vi "R1KSignalProcess.vi"(9 "error":errorcluster, 11 "LabVIEW Web Service":refnum<class "Web Service.lvclass">) -> (1 "error out":errorcluster)   [LabVIEW 2016]
uses:
  <vilib>/wsapi/Web Service.lvclass
  Controls/ISE.ctl
  Controls/Tri State Control.ctl
  Controls/ISE_CF.ctl
panel:
  out "R1Na":T1 {"Steady State?" items=["False", "True", "NaN", ""]}
  out "Carousel Array":dbl[][](array[numeric])
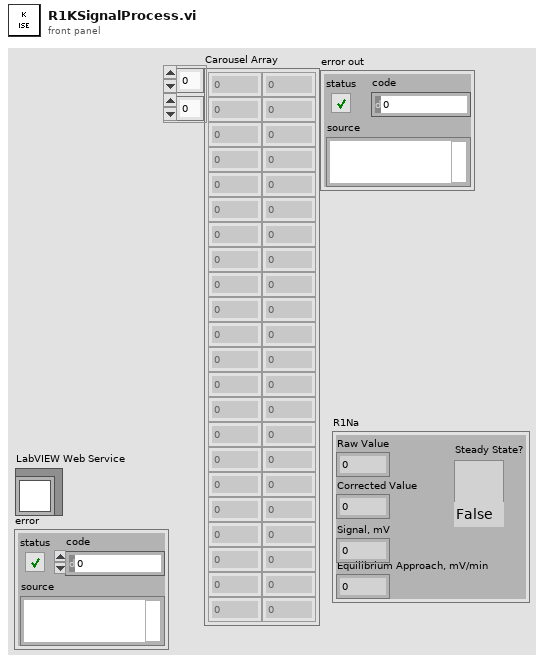
[diagram p1: front panel]
types:
  T1 = typedef "ISE.ctl" = cluster{"Raw Value":dbl, "Corrected Value":dbl, "Signal, mV":dbl, "Equilibrium Approach, mV/min":dbl, "Steady State?":T2}
  T2 = typedef "Tri State Control.ctl" = u16
  T3 = typedef "ISE_CF.ctl" = cluster{"Correction Factor":dbl, "Ion":string, "Correct For Ion?":bool}
  T4 = cluster{"Equil Approach Set point, mV/min":dbl, "Equil Approach dt, s":dbl, "Interference Correction Factors":T3[], "Detect Equilibrium?":bool, "Probe Intercept":dbl, "Probe Slope":dbl, "Baseline":dbl, "Detection Limit, M":dbl}
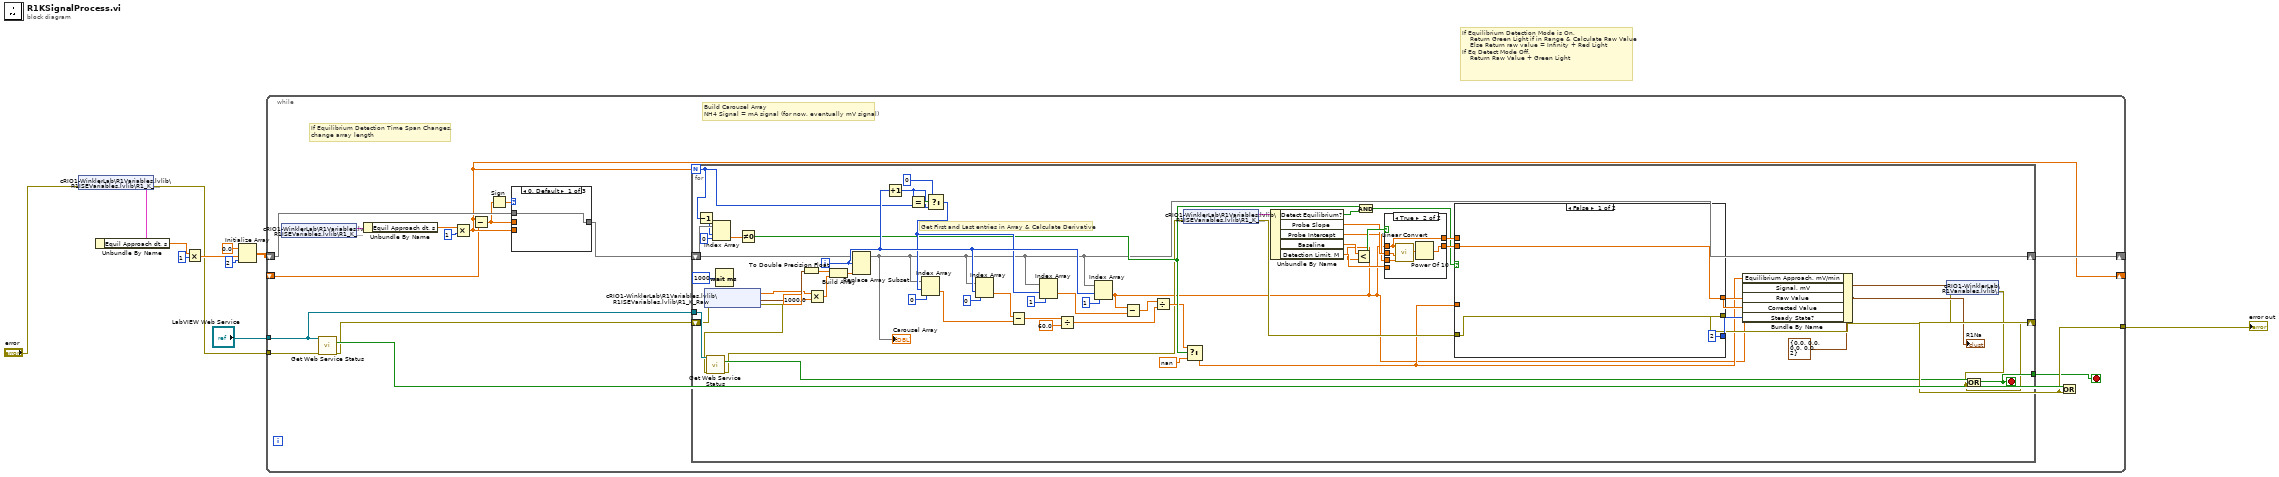
[diagram p0: block diagram]
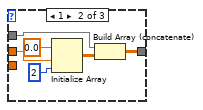
[diagram p2: hidden frame]
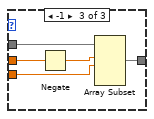
[diagram p3: hidden frame]
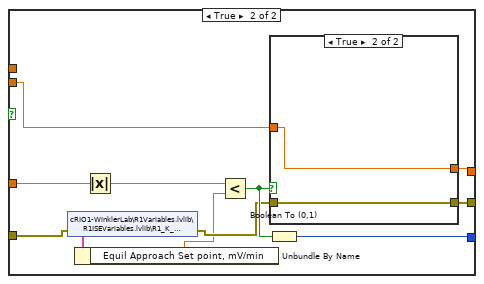
[diagram p5: hidden frame]
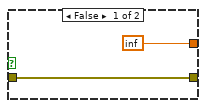
[diagram p6: hidden frame]
diagram:
  # "If Equilibrium Detection Mode is On, \n    Return Green Light if in Range & Calculate Raw Value\n    Else Return raw value = Infinity + Red Light\nIf Eq Detect Mode Off,\n    Return Raw Value + Green Light"
  n1 = shared-variable "cRIO1-WinklerLab\\R1Variables.lvlib\\R1ISEVariables.lvlib\\R1_K_SetParams"(error in="error") -> (w5:T4, error out=w1:errorcluster)
  n2 = Unbundle By Name(w5) -> ("Equil Approach dt, s"=w4:dbl)
  n3 = Multiply(x=w4, y=1) -> (x*y=w3:dbl)
  n4 = Initialize Array(0.0 ("element"), w3, 2 ("dimension size")) -> (w7:dbl[][])
  n5 = while {
    tunnel: "LabVIEW Web Service" -> [w27]
    tunnel: w1 -> [w17]
    shift-right: [w21] -> _
    shift-left: w7 -> [w24]
    shift-right: [w20] -> _
    shift-left: _ -> [w19]
    tunnel: [w16] -> w6
    stop <- w15 stop-if-true
    # "Build Carousel Array\nNH4 Signal = mA signal (for now, eventually mV signal)"
    # "If Equilibrium Detection Time Span Changes, \nchange array length"
    n6 = shared-variable "cRIO1-WinklerLab\\R1Variables.lvlib\\R1ISEVariables.lvlib\\R1_K_SetParams"() -> (w13:T4)  [unwired: 1 in, 1 out]
    n7 = call <vilib>:"Get Web Service Status.vi"("LabVIEW Web Service"=w27, "error in (no error)"=w17) -> ("service stopping?"=w18:bool, "error out"=w14:errorcluster)  [unwired: 11 in, 1 out]
    n8 = Unbundle By Name(w13) -> ("Equil Approach dt, s"=w12:dbl)
    n9 = Multiply(x=w12, y=1) -> (x*y=w20:dbl)
    n10 = Subtract(x=w20, y=w19) -> (x-y=w23:dbl)
    n11 = Sign(1:w23) -> (0:w25:dbl)
    n12 = case shown="0, Default" w25 {
      tunnel: w24 -> [w28 w32 w35]
      tunnel: w23 -> [_ w29 w37]
      tunnel: [w28 w30 w39] -> w22
      tunnel: w20 -> [_ _ w38]
      frame 0, Default {
      }
      frame 1 {
        n13 = Initialize Array(0.0 ("element"), w29, 2 ("dimension size")) -> (w31:dbl[][])
        n14 = Build Array (concatenate)(w32, w31) -> (w30:dbl[][])
      }
      frame -1 {
        n15 = Negate(x=w37) -> (-x=w36:dbl)
        n16 = Array Subset(array=w35, index (row)=w36, length (row)=w38) -> (w39:dbl[][])  [unwired: 2 in]
      }
    }
    n17 = for {
      N: w20 -> [w74]
      tunnel: w27 -> [w96]
      shift-right: [w68] -> w21
      shift-left: w22 -> [w80]
      shift-right: [w57] -> w16
      shift-left: w14 -> [w61]
      tunnel: [w60] -> w15
      i -> [w85]
      stop <- w60 stop-if-true
      # "Get First and Last entries in Array & Calculate Derivative"
      n18 = Decrement(x=w74) -> (x-1=w75:i32)
      n19 = shared-variable "cRIO1-WinklerLab\\R1Variables.lvlib\\R1ISEVariables.lvlib\\R1_K_Raw"(error in=w61) -> (w51:dbl, error out=w71:errorcluster, w72:timestamp)
      n20 = call <vilib>:"Get Web Service Status.vi"("LabVIEW Web Service"=w96, "error in (no error)"=w71) -> ("service stopping?"=w73:bool, "error out"=w56:errorcluster)  [unwired: 11 in, 1 out]
      n21 = Index Array(array=w80, index (row)=w75, index (col)=0 ("disabled index (col)")) -> (element=w78:dbl)
      n22 = Wait (ms)(milliseconds to wait=u32 1000) -> ()  [unwired: 1 out]
      n23 = Not Equal To 0?(x=w78) -> (x != 0?=w77:bool)
      n24 = To Double Precision Float(number=w72) -> (double precision float=w95:dbl)
      n25 = Multiply(x=w51, y=1000.0) -> (x*y=w50:dbl)
      n26 = Build Array(w95, w50) -> (w94:dbl[])
      n27 = Replace Array Subset(array=w80, new element=w94, index (row)=w85) -> (w68:dbl[][])  [unwired: 1 in]
      "Carousel Array" <- w68
      n28 = Increment(x=w85) -> (x+1=w48:i32)
      n29 = Equal?(x=w48, y=w74) -> (x = y?=w82:bool)
      n30 = Select(t=0, s=w82, f=w48) -> (s? t:f=w81:i32)
      n31 = Index Array(array=w68, index (row)=w81, index (col)=0 ("disabled index (col)")) -> (element=w87:dbl)
      n32 = Index Array(array=w68, index (row)=w85, index (col)=0 ("disabled index (col)")) -> (element=w83:dbl)
      n33 = Subtract(x=w83, y=w87) -> (x-y=w45:dbl)
      n34 = Index Array(array=w68, index (row)=w81, index (col)=1 ("disabled index (col)")) -> (element=w86:dbl)
      n35 = Divide(x=w45, y=60.0) -> (x/y=w44:dbl)
      n36 = Index Array(array=w68, index (row)=w85, index (col)=1 ("disabled index (col)")) -> (element=w40:dbl)
      n37 = Subtract(x=w40, y=w86) -> (x-y=w92:dbl)
      n38 = Divide(x=w92, y=w44) -> (x/y=w67:dbl)
      n39 = shared-variable "cRIO1-WinklerLab\\R1Variables.lvlib\\R1ISEVariables.lvlib\\R1_K_SetParams"(error in=w56) -> (w54:T4, error out=w55:errorcluster)
      n40 = Select(t=w67, s=w77, f=nan) -> (s? t:f=w42:dbl)
      n41 = Unbundle By Name(w54) -> ("Detect Equilibrium?"=w69:bool, "Probe Slope"=w65:dbl, "Probe Intercept"=w41:dbl, "Baseline"=w49:dbl, "Detection Limit, M"=w53:dbl)
      n42 = Less?(x=w49, y=w40) -> (x < y?=w66:bool)
      n43 = And(x=w77, y=w69) -> (x .and. y?=w62:bool)
      n44 = case shown="True" w66 {
        tunnel: w65 -> [_ w103]
        tunnel: w41 -> [_ w102]
        tunnel: w40 -> [w98 w101]
        tunnel: [w97 w100] -> w64
        tunnel: [w98 w101] -> w63
        tunnel: w53 -> [w97 _]
        frame False {
        }
        frame True {
          n45 = call "Linear Convert.vi"("Intercept"=w102, "Slope"=w103, "Signal"=w101) -> ("Result"=w99:dbl)  [unwired: 8 in]
          n46 = Power Of 10(x=w99) -> (10^x=w100:dbl)
        }
      }
      n47 = case shown="False" w62 {
        tunnel: [w106 w117] -> w70
        tunnel: w42 -> [_ w116]
        tunnel: [i16 2 w114] -> w84
        tunnel: w55 -> [w105 w110]
        tunnel: [w105 w111] -> w58
        tunnel: w64 -> [w106 w112]
        tunnel: w63 -> [_ _]
        frame False {
        }
        frame True {
          n48 = shared-variable "cRIO1-WinklerLab\\R1Variables.lvlib\\R1ISEVariables.lvlib\\R1_K_SetParams"(error in=w110) -> (w107:T4, error out=w109:errorcluster)
          n49 = Unbundle By Name(w107) -> ("Equil Approach Set point, mV/min"=w108:dbl)
          n50 = Absolute Value(x=w116) -> (abs(x)=w113:dbl)
          n51 = Less?(x=w113, y=w108) -> (x < y?=w115:bool)
          n52 = Boolean To (0,1)(Boolean=w115) -> (0, 1=w114:i16)
          n53 = case shown="True" w115 {
            tunnel: [inf w120] -> w117
            tunnel: w109 -> [w119 w121]
            tunnel: [w119 w121] -> w111
            tunnel: w112 -> [_ w120]
            frame False {
            }
            frame True {
            }
          }
        }
      }
      n54 = Bundle By Name(cluster=T1 {"Raw Value"=0.0, "Corrected Value"=0.0, "Signal, mV"=0.0, "Equilibrium Approach, mV/min"=0.0, "Steady State?"=2} ("R1NH4"), "Equilibrium Approach, mV/min"=w42, "Signal, mV"=w40, "Raw Value"=w70, "Corrected Value"=w70, "Steady State?"=w84) -> (w59:T1)
      "R1Na" <- w59
      n55 = shared-variable "cRIO1-WinklerLab\\R1Variables.lvlib\\R1ISEVariables.lvlib\\R1_K_ISE"(w59, error in=w58) -> (error out=w57:errorcluster)
      n56 = Or(x=w73, y=w57) -> (x .or. y?=w60:bool)
    }
    n57 = Or(x=w18, y=w16) -> ()  [unwired: 1 out]
  }
  "error out" <- w6
